vi "Select Platform UI.vi"(8 "error in (no error)":errorcluster, 11 "GVIWebProcessorApp in":refnum<class "GVIWebProcessorApp.lvclass">) -> (0 "error out":errorcluster, 1 "Cancelled":bool, 3 "Platform":string)   [LabVIEW 2020, in "PicoG-Processor.lvlib" / "GVIWebProcessorApp.lvclass"]
uses:
  GVIWebProcessorApp.lvclass
  GVIWebProcessorApp.lvclass/GVIWebProcessorApp.ctl
  Builds/picoG/ppl/PicoG-Core.lvlibp/TargetPluginManager/TargetPluginManager.lvclass
panel:
  in  "Cancel":bool
  in  "OK":bool
  in  "Select Platform":string(combo)
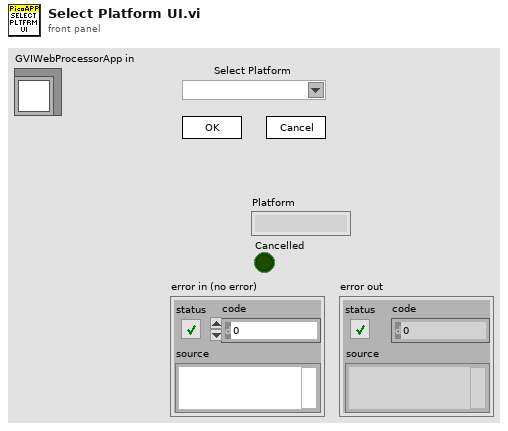
[diagram p1: front panel]
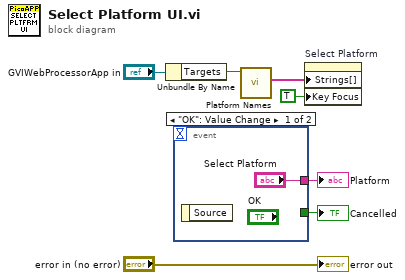
[diagram p0: block diagram]
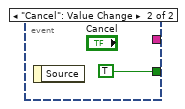
[diagram p2: hidden frame]
diagram:
  n1 = Unbundle By Name("GVIWebProcessorApp in") -> ("Targets"=w6:refnum<class "TargetPluginManager.lvclass">)
  n2 = event shown="[0] \"OK\": Value Change" {
    selector: _ -> [_ _]
    dyn-events: _ -> [_ _]
    timeout: _ -> [_ _]
    tunnel: ["Select Platform" _] -> w3
    tunnel: [_ TRUE] -> w2
    event "OK": Value Change {
      n3 = event-data() -> ()  [unwired: 1 in, 1 out]
    }
    event "Cancel": Value Change {
      n4 = event-data() -> ()  [unwired: 1 in, 1 out]
    }
  }
  "Platform" <- w3
  "Cancelled" <- w2
  n5 = call "Platform Names.vi"("TargetPluginManager in"=w6) -> ("Platforms"=w5:string[])  [unwired: 8 in, 2 out]
  n6 = property on="Select Platform" class="CmbBox"("Strings[]"=w5, "Key Focus"=TRUE) -> ()  [unwired: 2 in, 2 out]
  "error out" <- "error in (no error)"
